vi "TCP Initialize.vi"() -> (0 "error out":errorcluster, 1 "connection ID":refnum<k5>)   [LabVIEW 2018]
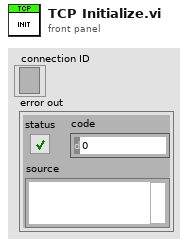
[diagram p1: front panel]
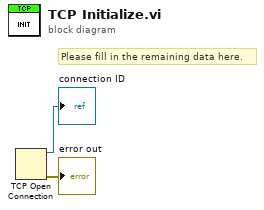
[diagram p0: block diagram]
diagram:
  # "Please fill in the remaining data here."
  n1 = TCP Open Connection() -> (connection ID=→"connection ID":refnum<k5>, error out=→"error out":errorcluster)  [unwired: 5 in]
